vi "getDatabase.vi"(8 "error in (no error)":errorcluster, 11 "CompiledList in":refnum<class "CompiledList.lvclass">) -> (0 "error out":errorcluster, 2 "deviceDataBase out":refnum<class "deviceDataBase.lvclass">, 3 "CompiledList out":refnum<class "CompiledList.lvclass">)   [LabVIEW 2009, in "Compiler.lvlib" / "CompiledList.lvclass"]
uses:
  CompiledList.lvclass
  DatabaseHelpers/DbConnection/DeviceDataBase/deviceDataBase.lvclass
  DatabaseHelpers.lvlib
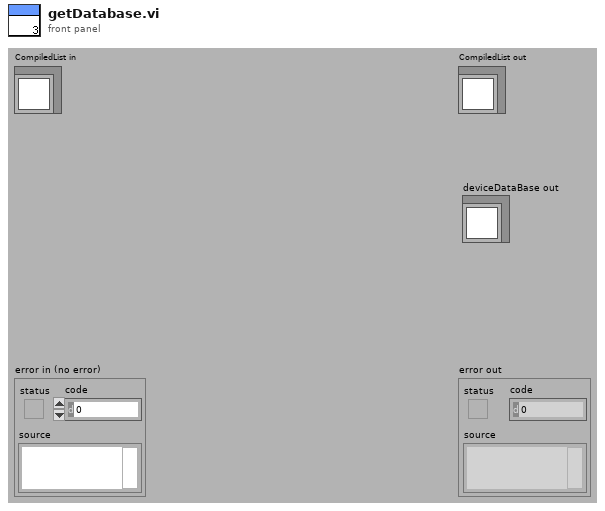
[diagram p1: front panel]
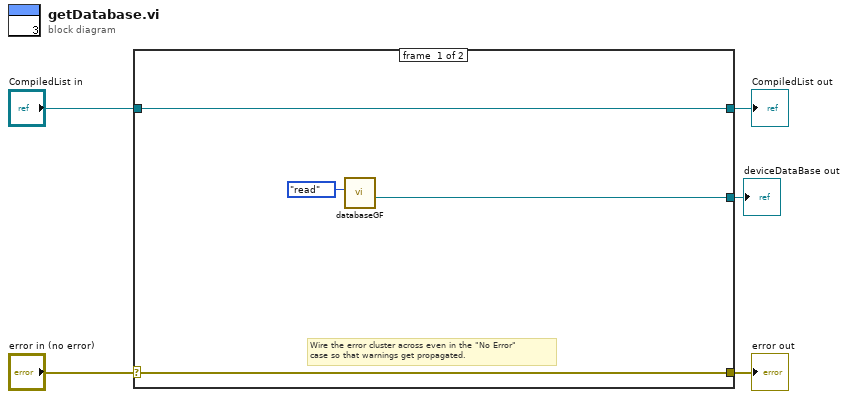
[diagram p0: block diagram]
diagram:
  n1 = case shown="No Error" "error in (no error)" {
    selector: "error in (no error)" -> [w8 w11]
    tunnel: [w8 w11] -> w4
    tunnel: [w9 w10] -> w2
    tunnel: "CompiledList in" -> [w9 w10]
    tunnel: [w6 _] -> w1
    frame #0 {
      # "Wire the error cluster across even in the \"No Error\"\ncase so that warnings get propagated."
      n2 = call "databaseGF.vi"("Enum"=enum16{"write", "read"}."read") -> ("deviceDataBase out"=w6:refnum<class "deviceDataBase.lvclass">)  [unwired: 10 in]
    }
    frame #1 {
    }
  }
  "error out" <- w4
  "CompiledList out" <- w2
  "deviceDataBase out" <- w1
